vi "fxpe_to_i64.vi"(1 "fxp64_32":fxp<+/-,64,32>) -> (0 "64bit integer":i64)   [LabVIEW 2018]
uses:
  <vilib>/rvi/FXPMathLib/FxpInterpret/XNode/nifxpmath_Interpret.xnode
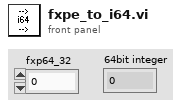
[diagram p1: front panel]
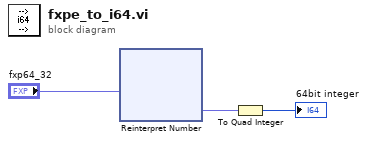
[diagram p0: block diagram]
diagram:
  n1 = xnode "Reinterpret Number"("x"="fxp64_32") -> ("y"=w2:fxp<+/-,64,64>)
  n2 = To Quad Integer(1:w2) -> (0:→"64bit integer":i64)
